vi "Test Parse Pattern.vi"() -> ()   [LabVIEW 2020]
uses:
  stream/URLPattern/URL Pattern Init.ctl
  stream/URLPattern/URLPattern.lvclass
panel:
  out "Pattern":T1
  in  "Pattern String":string
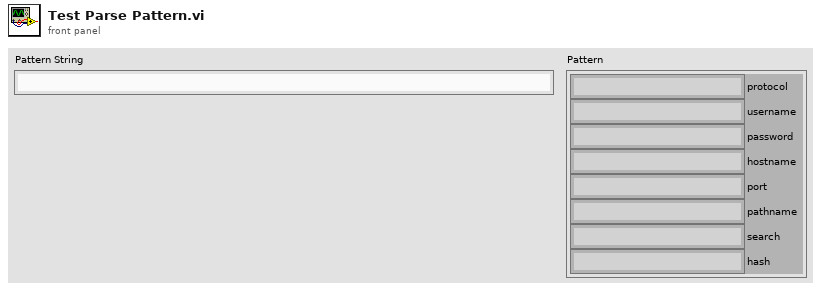
[diagram p1: front panel]
types:
  T1 = typedef "Stream.lvlib/URLPattern.lvclass/URL Pattern Init.ctl" = cluster{"protocol":string, "username":string, "password":string, "hostname":string, "port":string, "pathname":string, "search":string, "hash":string}
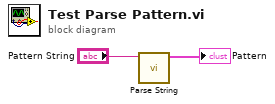
[diagram p0: block diagram]
diagram:
  n1 = call "Parse String.vi"("Pattern String"="Pattern String") -> ("Pattern"=→"Pattern":T1)  [unwired: 10 in]
